vi "TestStatusTableBuilder.vi"(0 "array":string[][](array[string]), 1 "Test Case Timeout":bool, 2 "STOP Button Pressed":bool, 3 "Test Case Target Reached":bool=TRUE, 5 "Test State":string="Ramping RPM", 7 "Test Status":string="Target Reached", 9 "Measurement":dbl=6000.0 format="%#_13g", 11 "Units":string="RPM") -> (4 "Table Control":string[][](table))   [LabVIEW 2026]
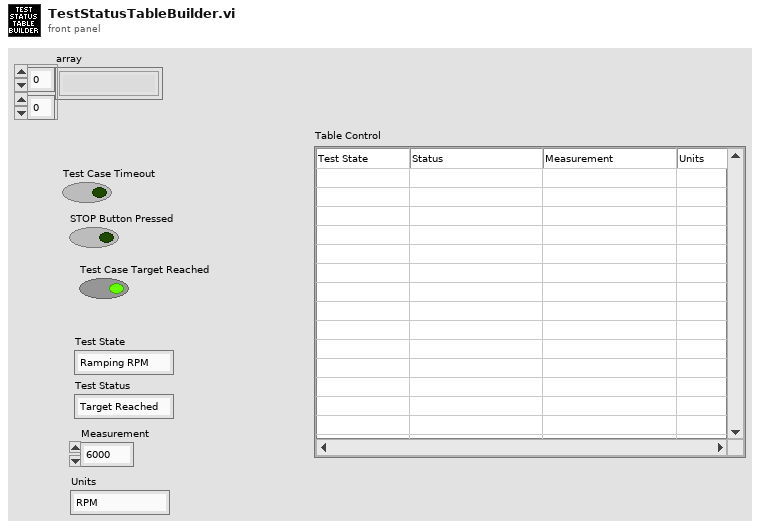
[diagram p1: front panel]
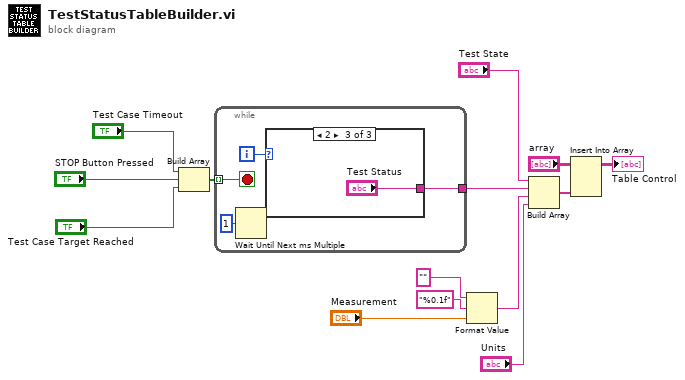
[diagram p0: block diagram]
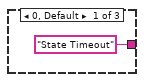
[diagram p2: hidden frame]
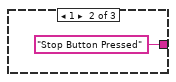
[diagram p3: hidden frame]
diagram:
  n1 = Build Array("Test Case Timeout", "STOP Button Pressed", "Test Case Target Reached") -> (w2:bool[])
  n2 = while {
    tunnel: w2 -> [w18] mode=indexing
    tunnel: [w16] -> w1
    i -> [w17]
    stop <- w18 stop-if-true
    n3 = Wait Until Next ms Multiple(millisecond multiple=u32 1) -> ()  [unwired: 1 out]
    n4 = case shown="2" w17 {
      tunnel: ["State Timeout" ("Test Status") "Stop Button Pressed" ("Test Status") "Test Status"] -> w16
      frame 0, Default {
      }
      frame 1 {
      }
      frame 2 {
      }
    }
  }
  n5 = Format Value(string ("")="", format string="%0.1f", value (0)="Measurement") -> (output string=w8:string)
  n6 = Build Array("Test State", w1, w8, "Units") -> (w6:string[])
  n7 = Insert Into Array(array="array", new element=w6) -> (→"Table Control":string[][])  [unwired: 2 in]
